vi "week01hello.vi"() -> ()   [LabVIEW 2021]
panel:
  in  "Slide":dbl(slide) scale=0.0..10.0
  out "Tank":dbl(slide) scale=0.0..10.0
  out "output 2":string
  out "output":string
  out "Boolean":bool
  in  "another input":string
  in  "AMP":dbl(knob) scale=0.0..10.0
  in  "input":string
  out "Numeric":dbl
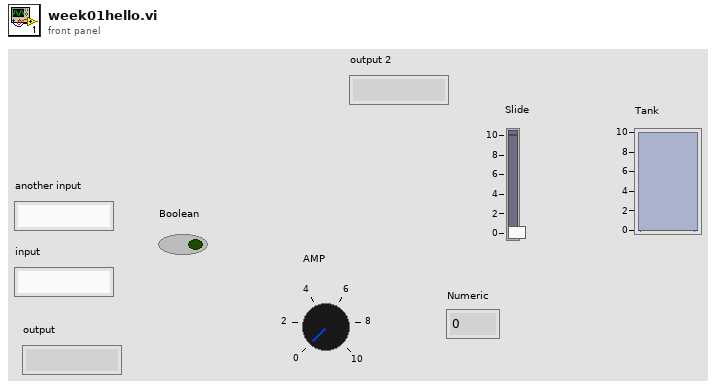
[diagram p1: front panel]
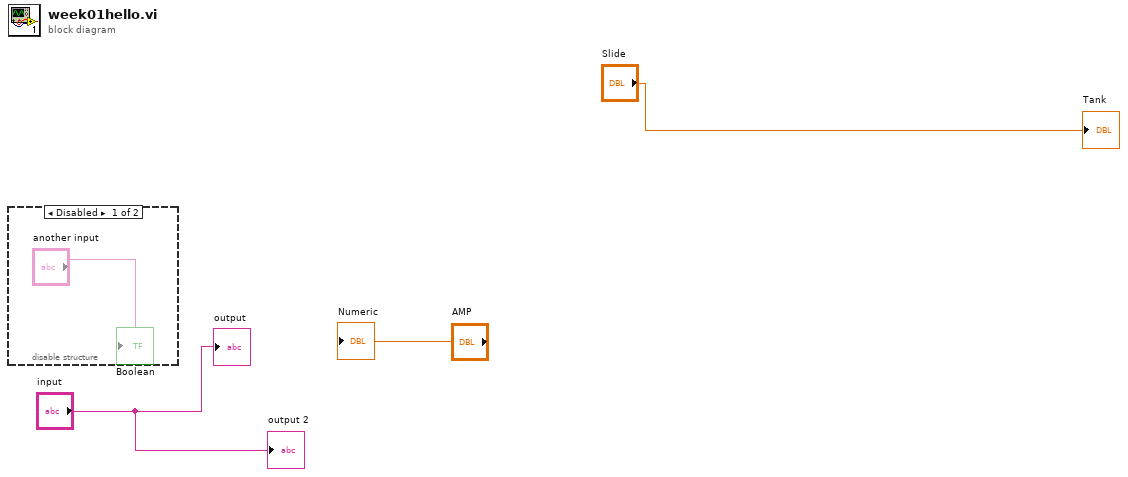
[diagram p0: block diagram]
diagram:
  n1 = disable-structure shown="Disabled" {
    frame Disabled {
      "Boolean" <- "another input"
    }
    frame Enabled {
    }
  }
  "Numeric" <- "AMP"
  "output" <- "input"
  "output 2" <- "input"
  "Tank" <- "Slide"
